vi "LoadConfig.vi"(8 "error in (no error)":errorcluster, 10 "config file path (Empty: use configured)":path, 11 "BASE in":refnum<class "BASE.lvclass">) -> (0 "error out":errorcluster, 3 "BASE out":refnum<class "BASE.lvclass">)   [LabVIEW 2019, in "BASE.lvlib" / "BASE.lvclass"]
uses:
  BASE.lvclass
  BASE.lvclass/BASE.ctl
  <userlib>/_OpenG.lib/file/file.llb/Convert File Extension (Path)__ogtk.vi
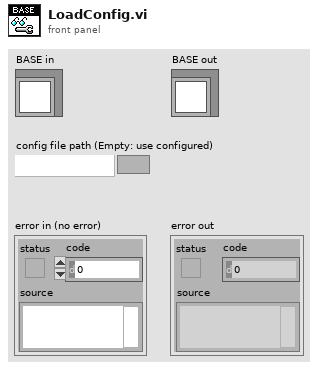
[diagram p1: front panel]
types:
  T1 = typedef "BASE.lvlib/BASE.lvclass/config--cluster.ctl" = cluster{"Config Path":path}
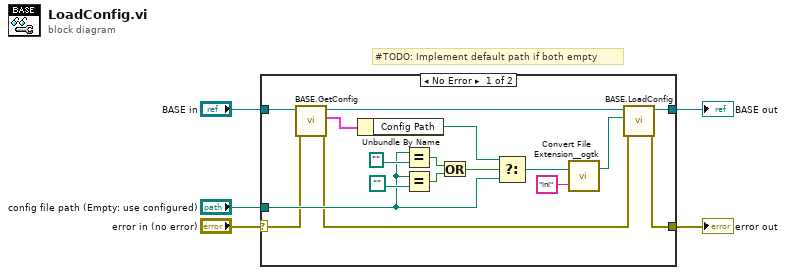
[diagram p0: block diagram]
diagram:
  # "#TODO: Implement default path if both empty"
  n1 = case shown="No Error" "error in (no error)" {
    selector: "error in (no error)" -> [w7 w23]
    tunnel: "BASE in" -> [w10 w24]
    tunnel: [w22 w24] -> w4
    tunnel: [w21 w23] -> w3
    tunnel: "config file path (Empty: use configured)" -> [w12 _]
    frame No Error {
      n2 = call "BASE.GetConfig.vi"("error in (no error)"=w7, "BASE in"=w10) -> ("error out"=w6:errorcluster, "Config"=w9:T1, "BASE out"=w8:refnum<class "BASE.lvclass">)  [unwired: 7 in]
      n3 = Unbundle By Name(w9) -> ("Config Path"=w18:path)
      n4 = Equal?(x=w12, y=path "") -> (x = y?=w16:bool)
      n5 = Equal?(x=w12, y=path "") -> (x = y?=w15:bool)
      n6 = Or(x=w16, y=w15) -> (x .or. y?=w17:bool)
      n7 = Select(t=w18, s=w17, f=w12) -> (s? t:f=w11:path)
      n8 = call-poly <userlib>:"Convert File Extension__ogtk.vi"("new ending (none)"="ini", "file name"=w11) -> ("new filename"=w19:path)  [unwired: 1 out]
      n9 = call-dynamic "BASE.LoadConfig.vi"("error in (no error)"=w6, "config file path"=w19, "BASE in"=w8) -> ("error out"=w21:errorcluster, "BASE out"=w22:refnum<class "BASE.lvclass">)  [unwired: 7 in]
    }
    frame Error {
    }
  }
  "error out" <- w3
  "BASE out" <- w4
